vi "dydx circle.vi"(4 "count?":bool, 6 "Desired X in":dbl, 7 "X Position":dbl, 9 "Y Position":dbl, 10 "Desired Y in":dbl, 11 "Allowable Error 2":dbl) -> (1 "X Control":dbl, 2 "ChangeState":i32, 3 "Y Control":dbl)   [LabVIEW 2015]
uses:
  <vilib>/addons/control/pid/NI_PID_pid.lvlib
  <vilib>/addons/control/pid/pid.llb/PID (DBL).vi
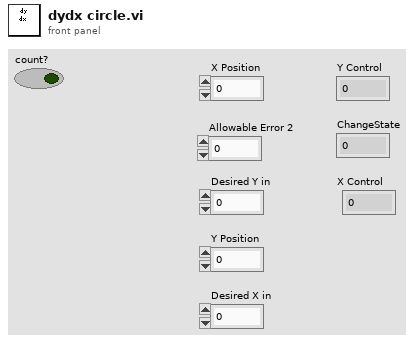
[diagram p1: front panel]
types:
  T1 = cluster{"proportional gain (Kc)":dbl, "integral time (Ti, min)":dbl, "derivative time (Td, min)":dbl}
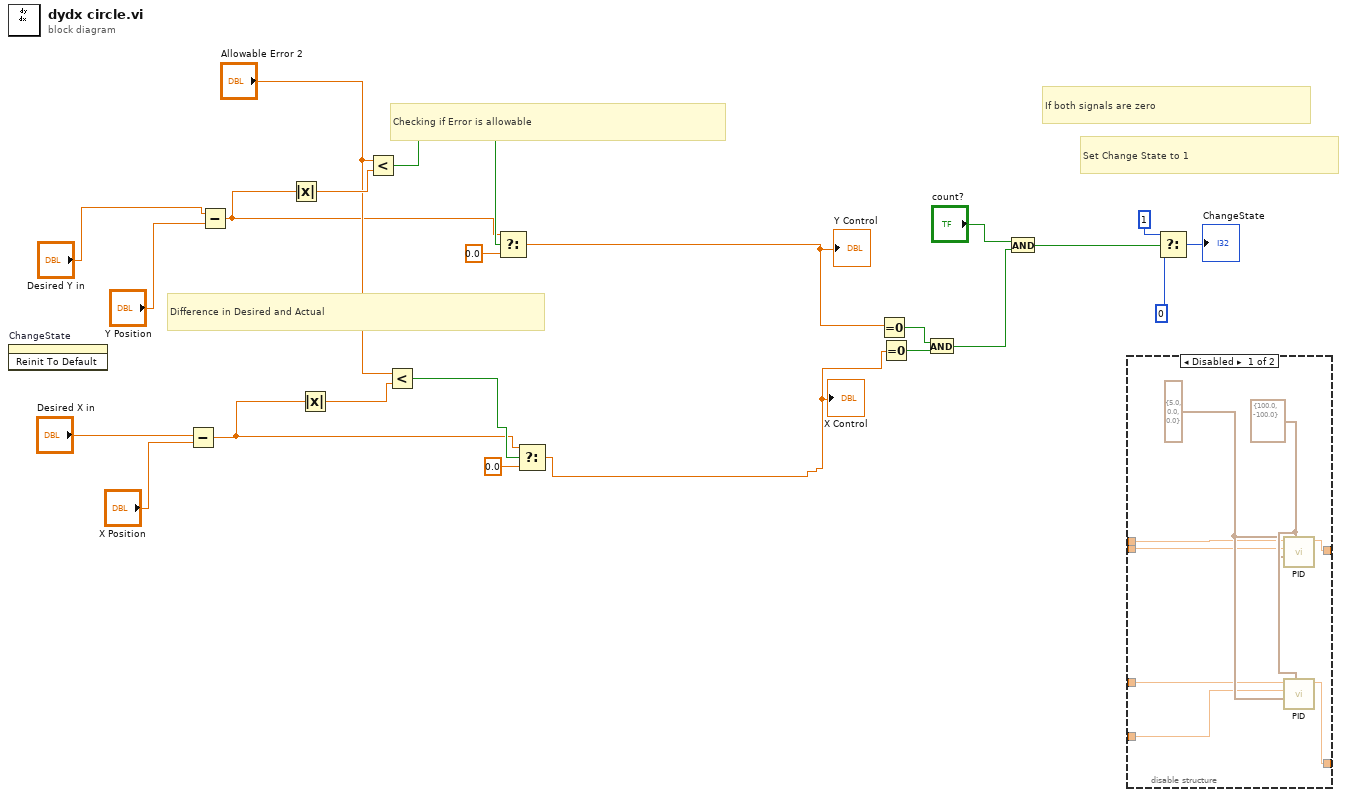
[diagram p0: block diagram]
diagram:
  # "Set Change State to 1"
  # "If both signals are zero"
  # "Checking if Error is allowable"
  # "Difference in Desired and Actual"
  n1 = invoke on="ChangeState" class="DigNum (strict)" method="Reinit To Default"() -> ()  [unwired: 3 in, 3 out]
  n2 = Subtract(x="Desired X in", y="X Position") -> (x-y=w4:dbl)
  n3 = Subtract(x="Desired Y in", y="Y Position") -> (x-y=w5:dbl)
  n4 = Absolute Value(x=w5) -> (abs(x)=w15:dbl)
  n5 = Absolute Value(x=w4) -> (abs(x)=w17:dbl)
  n6 = Less?(x="Allowable Error 2", y=w15) -> (x < y?=w14:bool)
  n7 = Less?(x="Allowable Error 2", y=w17) -> (x < y?=w13:bool)
  n8 = Select(t=w5, s=w14, f=0.0) -> (s? t:f=w11:dbl)
  "Y Control" <- w11
  n9 = Select(t=w4, s=w13, f=0.0) -> (s? t:f=w10:dbl)
  "X Control" <- w10
  n10 = Equal To 0?(x=w11) -> (x = 0?=w19:bool)
  n11 = Equal To 0?(x=w10) -> (x = 0?=w20:bool)
  n12 = And(x=w19, y=w20) -> (x .and. y?=w3:bool)
  n13 = And(x="count?", y=w3) -> (x .and. y?=w1:bool)
  n14 = disable-structure shown="Disabled" {
    disable-tunnel: _ -> [w29 _]
    disable-tunnel: _ -> [w28 _]
    disable-tunnel: _ -> [w27 _]
    disable-tunnel: _ -> [w26 _]
    disable-tunnel: [w25 _] -> _
    disable-tunnel: [w24 _] -> _
    frame Disabled {
      w30 = T1 {"proportional gain (Kc)"=5.0, "integral time (Ti, min)"=0.0, "derivative time (Td, min)"=0.0} ("PID gains")
      w31 = cluster{"output high":dbl, "output low":dbl} {"output high"=100.0, "output low"=-100.0} ("output range")
      n15 = call-poly <vilib>:"PID.vi"("output range"=w31, "PID gains"=w30, "process variable"=w27, "setpoint"=w26) -> ("output"=w25:dbl)  [unwired: 6 in, 1 out]
      n16 = call-poly <vilib>:"PID.vi"("output range"=w31, "PID gains"=w30, "process variable"=w29, "setpoint"=w28) -> ("output"=w24:dbl)  [unwired: 6 in, 1 out]
    }
    frame Enabled {
    }
  }
  n17 = Select(t=1, s=w1, f=0) -> (s? t:f=→"ChangeState":i32)
